vi "Get Graph Bounds.vi"(0 "eye scan point iterator":refnum<class "niHighSpeedSerial N Point Eye Scan Point Iterator v1 Host.lvclass">, 11 "error in":errorcluster) -> (4 "eye scan point iterator out":refnum<class "niHighSpeedSerial N Point Eye Scan Point Iterator v1 Host.lvclass">, 6 "x scale.range":T2, 8 "x scale.offset and multiplier":T1, 10 "y scale.range":T2, 14 "y scale.offset and multiplier":T1, 15 "error out":errorcluster)   [LabVIEW 2014, in "niHighSpeedSerial N Point Eye Scan Point Iterator v1 Host.lvclass"]
doc: "Returns the x, y, and z bounds to properly format an Intensity Graph given the configuration of the Point Iterator.\n\n<B>Input Parameters</B>\n\n<B>eye scan point iterator</B> is the incoming wire for the Eye Scan Point Iterator class object\n\n<B>error in</B> describes error conditions that occur before this node runs. This input provides standard 'error in' functionality.\n\n<B>Output Parameters</B>\n\n<B>eye scan point iterator out</B> is the outgoing wire for the Eye Scan Point Iterator class object\n\n<B>x scale.range</B> is the range for the x scale.\n\n<B>x scale.range.Minimum</B> is the minimum value for the x scale's range.\n\n<B>x scale.range.Maximum</B> is the maximum value for the x scale's range.\n\n<B>x scale.range.Increment</B> is the increment for the x scale's range.\n\n<B>x scale.range.Minor Increment</B> is the minor increment value for the x scale's range.\n\n<B>x scale.range.Start</B> is the start value for the x scale's range\n\n<B>x scale.offset and multiplier</B> is the offset and multiplier for the x scale's range.\n\n<B>x scale.offset and multiplier.Offset</B> is the offset for the x scale's range.\n\n<B>x scale.offset and multiplier.Multiplier</B> is the multiplier for the x scale's range.\n\n<B>y scale.range</B> is the range for the y scale.\n\n<B>y scale.range.Minimum</B> is the minimum for the y scale's range.\n\n<B>y scale.range.Maximum</B> is the maximum for the y scale's range.\n\n<B>y scale.range.Increment</B> is the increment for the y scale's range.\n\n<B>y scale.range.Minor Increment</B> is the minor increment for the y scale's range.\n\n<B>y scale.range.Start</B> is the start for the y scale's range.\n\n<B>y scale.offset and multiplier</B> is the offset and multiplier for the y scale's range.\n\n<B>y scale.offset and multiplier.Offset</B> is the offset for the y scale's range.\n\n<B>y scale.offset and multiplier.Multiplier</B> is the multiplier for the y scale's range.\n\n<B>error out</B> contains error information. This output provides standard 'error out' functionality."
uses:
  <instrlib>/niHighSpeedSerial/Eye Scan/v1/Host/Impl/N Pt Iter/niHighSpeedSerial N Point Eye Scan Point Iterator v1 Host.lvclass
  <vilib>/Utility/miscctls.llb/LVRangeTypeDef.ctl
  <vilib>/Utility/miscctls.llb/LVOffsetAndMultiplierTypeDef.ctl
  <vilib>/Utility/error.llb/Error Cluster From Error Code.vi
  <vilib>/ErrorRing/Error Ring.xnode
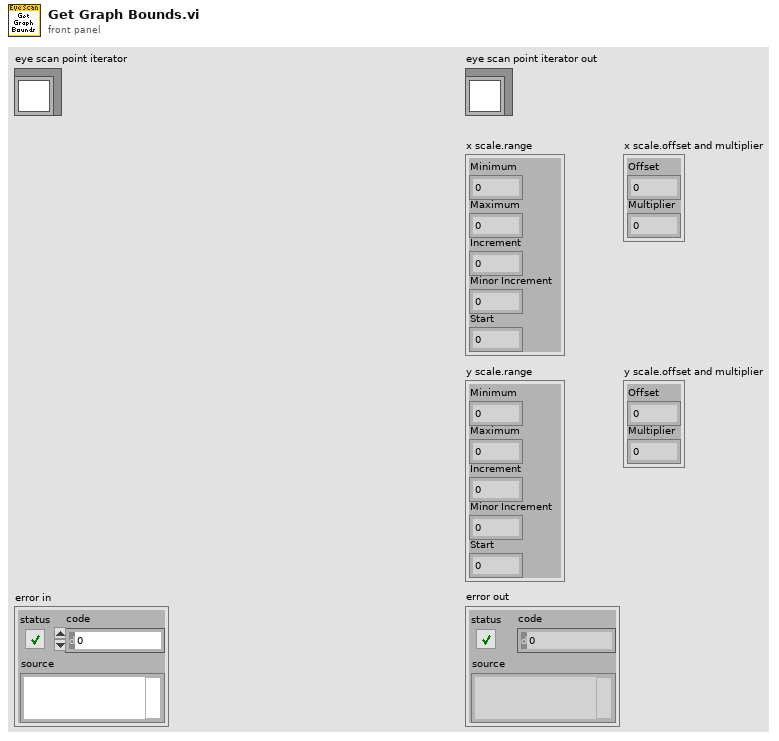
[diagram p1: front panel]
types:
  T1 = typedef "LVOffsetAndMultiplierTypeDef.ctl" = cluster{"Offset":dbl, "Multiplier":dbl}
  T2 = typedef "LVRangeTypeDef.ctl" = cluster{"Minimum":dbl, "Maximum":dbl, "Increment":dbl, "Minor Increment":dbl, "Start":dbl}
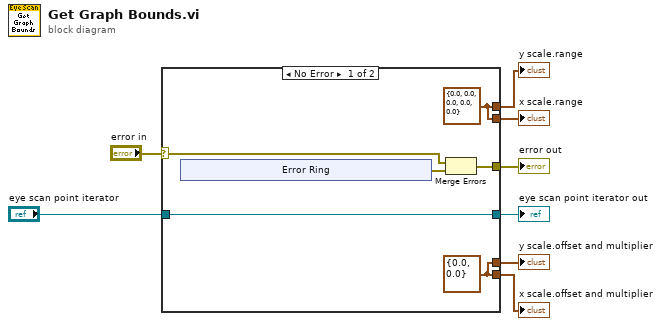
[diagram p0: block diagram]
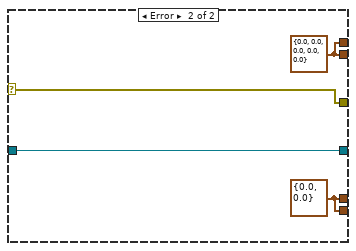
[diagram p2: hidden frame]
diagram:
  n1 = case shown="No Error" "error in" {
    selector: "error in" -> [w11 w22]
    tunnel: [w10 w22] -> w7
    tunnel: [w14 w21] -> w6
    tunnel: "eye scan point iterator" -> [w14 w21]
    tunnel: [w13 w20] -> w4
    tunnel: [w13 w20] -> w3
    tunnel: [w12 w19] -> w2
    tunnel: [w12 w19] -> w1
    frame No Error {
      w12 = T1 {"Offset"=0.0, "Multiplier"=0.0} ("X Scale.Offset and Multiplier")
      w13 = T2 {"Minimum"=0.0, "Maximum"=0.0, "Increment"=0.0, "Minor Increment"=0.0, "Start"=0.0} ("X Scale.Range")
      n2 = xnode "Error Ring"() -> ("error out"=w9:errorcluster)
      n3 = Merge Errors(w11, w9) -> (w10:errorcluster)
    }
    frame Error {
      w19 = T1 {"Offset"=0.0, "Multiplier"=0.0} ("X Scale.Offset and Multiplier")
      w20 = T2 {"Minimum"=0.0, "Maximum"=0.0, "Increment"=0.0, "Minor Increment"=0.0, "Start"=0.0} ("X Scale.Range")
    }
  }
  "error out" <- w7
  "eye scan point iterator out" <- w6
  "x scale.range" <- w4
  "y scale.range" <- w3
  "x scale.offset and multiplier" <- w1
  "y scale.offset and multiplier" <- w2
